vi "Ask for Connected Devices.vi"(8 "error in (no error)":errorcluster, 10 "Delay between send and receive [ms]":u32, 11 "Communicator in":refnum<class "Communicator.lvclass">) -> (0 "error out":errorcluster, 3 "appended array":string[](array[string]))   [LabVIEW 2023, in "DeviceManager.lvlib"]
uses:
  DeviceManager.lvlib
  Classes/Communicator/Communicator.lvclass
panel:
  # "Connector Pane"
  # "Locals"
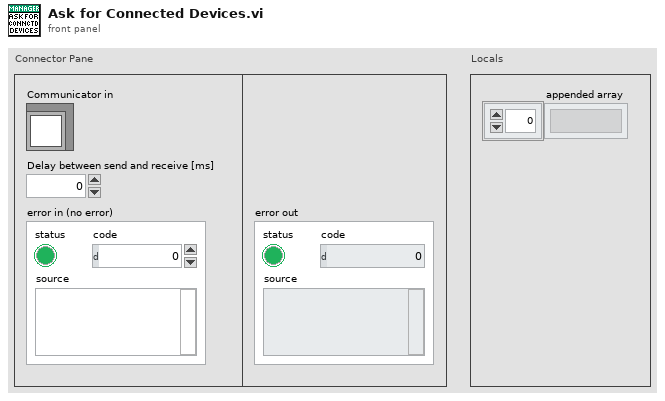
[diagram p1: front panel]
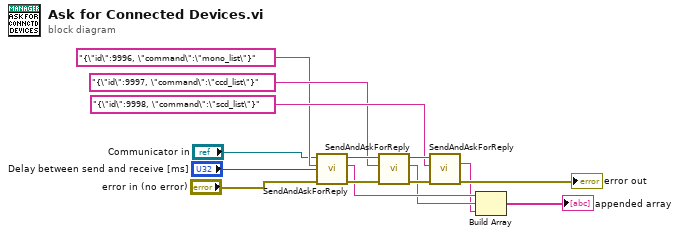
[diagram p0: block diagram]
diagram:
  n1 = call-dynamic "SendAndAskForReply.vi"("error in (no error)"="error in (no error)", "timeout for receiving data [ms]"="Delay between send and receive [ms]", "String to be sent"="{\"id\":9996, \"command\":\"mono_list\"}", "Communicator in"="Communicator in") -> ("error out"=w13:errorcluster, "Data"=w4:string, "Communicator out"=w9:refnum<class "Communicator.lvclass">)  [unwired: 5 in]
  n2 = call-dynamic "SendAndAskForReply.vi"("error in (no error)"=w13, "String to be sent"="{\"id\":9997, \"command\":\"ccd_list\"}", "Communicator in"=w9) -> ("error out"=w14:errorcluster, "Data"=w3:string, "Communicator out"=w11:refnum<class "Communicator.lvclass">)  [unwired: 6 in]
  n3 = call-dynamic "SendAndAskForReply.vi"("error in (no error)"=w14, "String to be sent"="{\"id\":9998, \"command\":\"scd_list\"}", "Communicator in"=w11) -> ("error out"=→"error out":errorcluster, "Data"=w2:string)  [unwired: 6 in, 1 out]
  n4 = Build Array(w4, w3, w2) -> (→"appended array":string[])
